vi "Int.vi"(11 "reset":bool) -> (0 "error out":errorcluster, 3 "Vo":refnum<visa-resource-name>)   [LabVIEW 2016]
panel:
  in  "error in (no error)":errorcluster
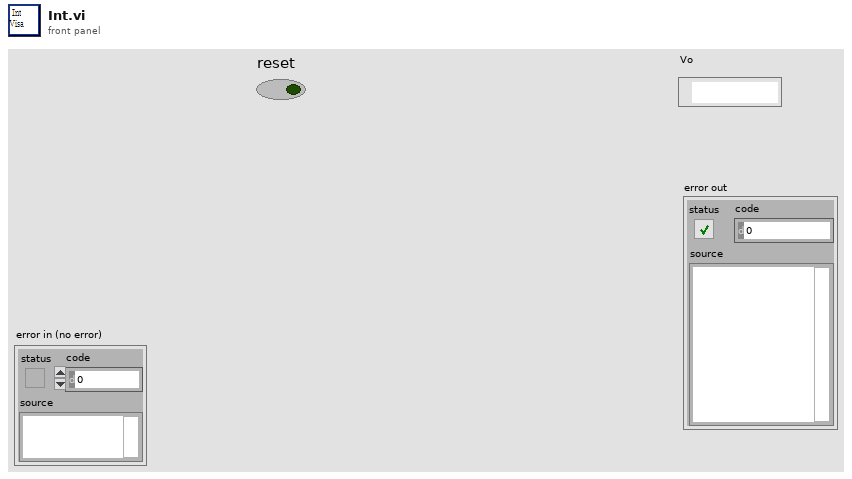
[diagram p1: front panel]
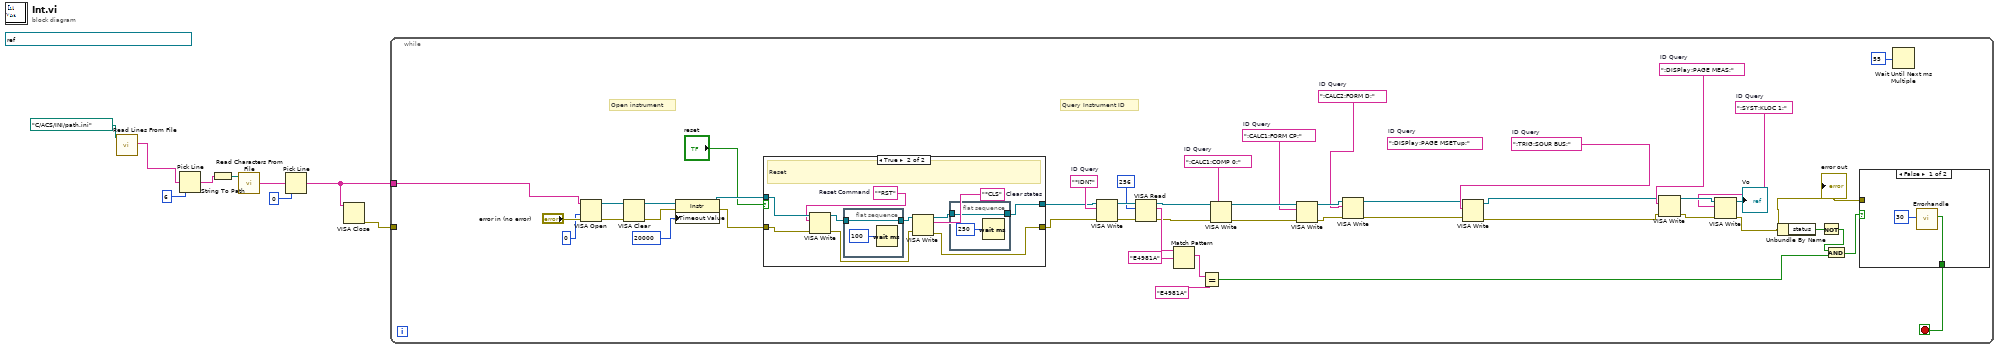
[diagram p0: block diagram]
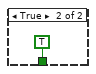
[diagram p3: hidden frame]
diagram:
  (unwired) refnum<visa-resource-name> "USB0::0x0957::0x0F09::MY48310636::INSTR" ("VISA resource name 2")
  n1 = call <vilib>:"Read Lines From File.vi"("file path (dialog if empty)"=path "C:/ACS/INI/path.ini") -> ("line string"=w5:string)  [unwired: 5 in, 3 out]
  n2 = Pick Line(multi-line string=w5, line index=6) -> (output string=w7:string)  [unwired: 1 in]
  n3 = String To Path(string=w7) -> (path=w6:path)
  n4 = call <vilib>:"Read Characters From File.vi"("file path (dialog if empty)"=w6) -> ("character string"=w4:string)  [unwired: 5 in, 3 out]
  n5 = Pick Line(multi-line string=w4, line index=0) -> (output string=w1:string)  [unwired: 1 in]
  n6 = VISA Close(VISA resource name=w1) -> (error out=w2:errorcluster)  [unwired: 1 in]
  n7 = while {
    tunnel: w1 -> [w38]
    tunnel: w2 -> [_]
    stop <- w39 stop-if-true
    w17 = ":TRIG:SOUR BUS;"  # ID Query
    (unwired) ":DISPlay:PAGE MSETup;"  # ID Query
    w21 = ":SYST:KLOC 1;"  # ID Query
    w25 = ":DISPlay:PAGE MEAS;"  # ID Query
    w26 = ":CALC2:FORM D;"  # ID Query
    w27 = ":CALC1:FORM CP;"  # ID Query
    w36 = ":CALC1:COMP 0;"  # ID Query
    w44 = "*IDN?"  # ID Query
    # "Query Instrument ID"
    # "Open instrument"
    n8 = VISA Open(access mode=u32 0, error in (no error)="error in (no error)", VISA resource name=w38) -> (VISA resource name=w53:refnum<visa-resource-name>, error out=w52:errorcluster)  [unwired: 2 in]
    n9 = VISA Clear(VISA resource name=w53, error in (no error)=w52) -> (VISA resource name out=w51:refnum<visa-resource-name>, error out=w50:errorcluster)
    n10 = property class="Instr"(reference=w51, error in=w50, "General Settings:Timeout Value"=u32 20000) -> (reference out=w13:refnum<visa-resource-name>, error out=w11:errorcluster)
    n11 = case shown="True" "reset" {
      tunnel: [w58 w63] -> w14
      tunnel: w13 -> [w58 w68]
      tunnel: [w57 w61] -> w12
      tunnel: w11 -> [w57 w60]
      frame False {
      }
      frame True {
        w59 = "*CLS"  # Clear states
        w67 = "*RST"  # Reset Command
        # "Reset"
        n12 = VISA Write(VISA resource name=w68, write buffer=w67, error in (no error)=w60) -> (VISA resource name out=w65:refnum<visa-resource-name>, error out=w62:errorcluster)  [unwired: 1 out]
        n13 = flat-sequence {
          tunnel: [w71] -> w66
          tunnel: w65 -> [w71]
          frame #0 {
            n14 = Wait (ms)(milliseconds to wait=u32 100) -> ()  [unwired: 1 out]
          }
        }
        n15 = VISA Write(VISA resource name=w66, write buffer=w59, error in (no error)=w62) -> (VISA resource name out=w64:refnum<visa-resource-name>, error out=w61:errorcluster)  [unwired: 1 out]
        n16 = flat-sequence {
          tunnel: [w69] -> w63
          tunnel: w64 -> [w69]
          frame #0 {
            n17 = Wait (ms)(milliseconds to wait=u32 250) -> ()  [unwired: 1 out]
          }
        }
      }
    }
    n18 = VISA Write(VISA resource name=w14, write buffer=w44, error in (no error)=w12) -> (VISA resource name out=w48:refnum<visa-resource-name>, error out=w47:errorcluster)  [unwired: 1 out]
    n19 = VISA Read(VISA resource name=w48, byte count=u32 256, error in (no error)=w47) -> (VISA resource name out=w34:refnum<visa-resource-name>, read buffer=w49:string, error out=w35:errorcluster)  [unwired: 1 out]
    n20 = Match Pattern(string=w49, regular expression="E4981A") -> (match substring=w42:string)  [unwired: 1 in, 3 out]
    n21 = Equal?(x=w42, y="E4981A") -> (x = y?=w40:bool)
    n22 = VISA Write(VISA resource name=w34, write buffer=w36, error in (no error)=w35) -> (VISA resource name out=w31:refnum<visa-resource-name>, error out=w30:errorcluster)  [unwired: 1 out]
    n23 = VISA Write(VISA resource name=w31, write buffer=w27, error in (no error)=w30) -> (VISA resource name out=w28:refnum<visa-resource-name>, error out=w29:errorcluster)  [unwired: 1 out]
    n24 = VISA Write(VISA resource name=w28, write buffer=w26, error in (no error)=w29) -> (VISA resource name out=w16:refnum<visa-resource-name>, error out=w15:errorcluster)  [unwired: 1 out]
    n25 = VISA Write(VISA resource name=w16, write buffer=w17, error in (no error)=w15) -> (VISA resource name out=w19:refnum<visa-resource-name>, error out=w18:errorcluster)  [unwired: 1 out]
    n26 = VISA Write(VISA resource name=w19, write buffer=w25, error in (no error)=w18) -> (VISA resource name out=w22:refnum<visa-resource-name>, error out=w24:errorcluster)  [unwired: 1 out]
    n27 = VISA Write(VISA resource name=w22, write buffer=w21, error in (no error)=w24) -> (VISA resource name out=→"Vo":refnum<visa-resource-name>, error out=w23:errorcluster)  [unwired: 1 out]
    "error out" <- w23
    n28 = Unbundle By Name(w23) -> ("status"=w33:bool)
    n29 = Not(x=w33) -> (.not. x?=w32:bool)
    n30 = And(x=w32, y=w40) -> (x .and. y?=w43:bool)
    n31 = case shown="False" w43 {
      tunnel: [w74 TRUE ("cancel 2")] -> w39
      tunnel: w23 -> [_ _]
      frame False {
        n32 = call "Errorhandle.vi"("message"=30) -> ("cancel 2"=w74:bool)  [unwired: 17 in, 1 out]
      }
      frame True {
      }
    }
    n33 = Wait Until Next ms Multiple(millisecond multiple=u32 55) -> ()  [unwired: 1 out]
  }
